vi "FPGA_DAQ_FixedPoint.vi"() -> ()   [LabVIEW 2019]
doc: "This VI provides a template for customizing a waveform acquisition using delta-sigma based NI C Series analog input smodules."
uses:
  <vilib>/LabVIEW Targets/FPGA/cRIO/shared/nicrio_ModuleControls/nicrio_cRIO-9219_ConversionTime.ctl
  <vilib>/rvi/Emulation/niFpgaSctlEmulationGetInTimedLoop.vi
  <vilib>/LabVIEW Targets/FPGA/cRIO/shared/nicrio_DsaDataRateApi/_nicrio_9225GetDataRate131.vi
  <vilib>/LabVIEW Targets/FPGA/cRIO/shared/nicrio_DsaDataRateApi/_nicrio_9234GetDataRate131.vi
  <vilib>/rvi/Emulation/niFpgaProcessEmulError.vi
  <vilib>/rvi/eio/common/nirviEmuTemplatePropertySet_errors.vi
  <vilib>/rvi/eio/common/nirviEmuTemplateMethod_errors.vi
  <vilib>/rvi/Emulation/niFpgaGetClockAttributes.vi
  <vilib>/rvi/Emulation/niFpgaEmulationReportErrorSimple.vi
  <vilib>/rvi/Emulation/niFpgaCriticalErrorInLSC.vi
  <vilib>/rvi/interface/RandomDataEmulation/niFpgaRandomDataHandleErrors.vi
  <vilib>/eio/EIOPropertyNode/EIOPropertyNode.xnode
  <vilib>/LabVIEW Targets/FPGA/cRIO/shared/nicrio_ModuleControls/nicrio_cRIO-9225_DataRatesRing.ctl
  <vilib>/LabVIEW Targets/FPGA/cRIO/shared/nicrio_ModuleControls/nicrio_cRIO-9234_DataRatesRing2.ctl
  <vilib>/eio/EIONode/EIONode.xnode
  <vilib>/rvi/DataTransferAndStorage/Container/XNode/niFpgaContainer.xnode
  <vilib>/rvi/interface/RandomDataEmulation/nirviRandomDataFpgaReadWriteTemplate.vi
  <vilib>/rvi/eio/common/nirviEmuTemplatePropertyGet_errors.vi
  <vilib>/rvi/eio/common/nirviEmuTemplatePropertyGet_noerrors.vi
  <vilib>/rvi/eio/common/nirviEmuTemplatePropertySet_noerrors.vi
panel:
  in  "Measurements per cycle":i16
  out "StopGeral":bool
  out "CJC1":fxp<+/-,32,-1>
  out "CJC0":fxp<+/-,32,-1>
  out "Temp3":fxp<+,32,14>
  out "Temp2":fxp<+,32,14>
  out "Temp1":fxp<+/-,32,-1>
  out "Temp0":fxp<+/-,32,-1>
  out "Ten oclk mult":u32
  out "Ten oclk div":u32
  out "Ten oclk freq":u32
  out "Vib oclk mult":u32
  out "Vib oclk div":u32
  out "Vib oclk freq":u32
  out "Acq Loop uS":u32
  out "FPGA Error":errorcluster
  out "Module Underflow":bool
  out "Finished":bool
  out "First Read":bool
  out "DMA FIFO Full":bool
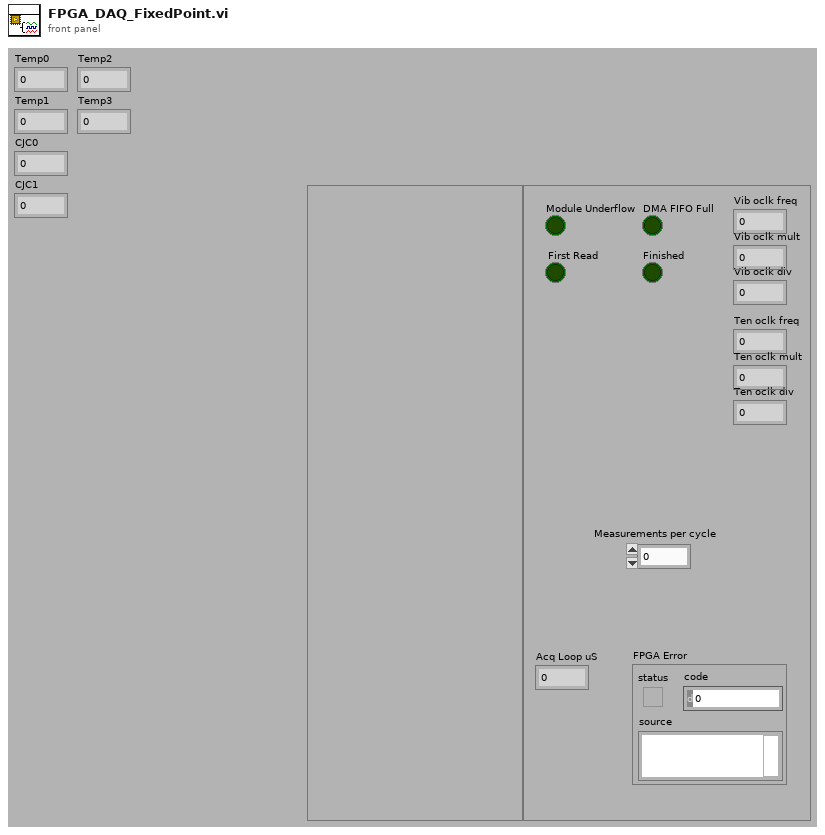
[diagram p1: front panel]
types:
  T1 = typedef "nicrio_cRIO-9219_ConversionTime.ctl" = enum8{"High Speed", "Best 60 Hz Rejection", "Best 50 Hz Rejection", "High Resolution"}
  T2 = typedef "nicrio_cRIO-9234_DataRatesRing2.ctl" = u8
  T3 = typedef "nicrio_cRIO-9225_DataRatesRing2.ctl" = u8
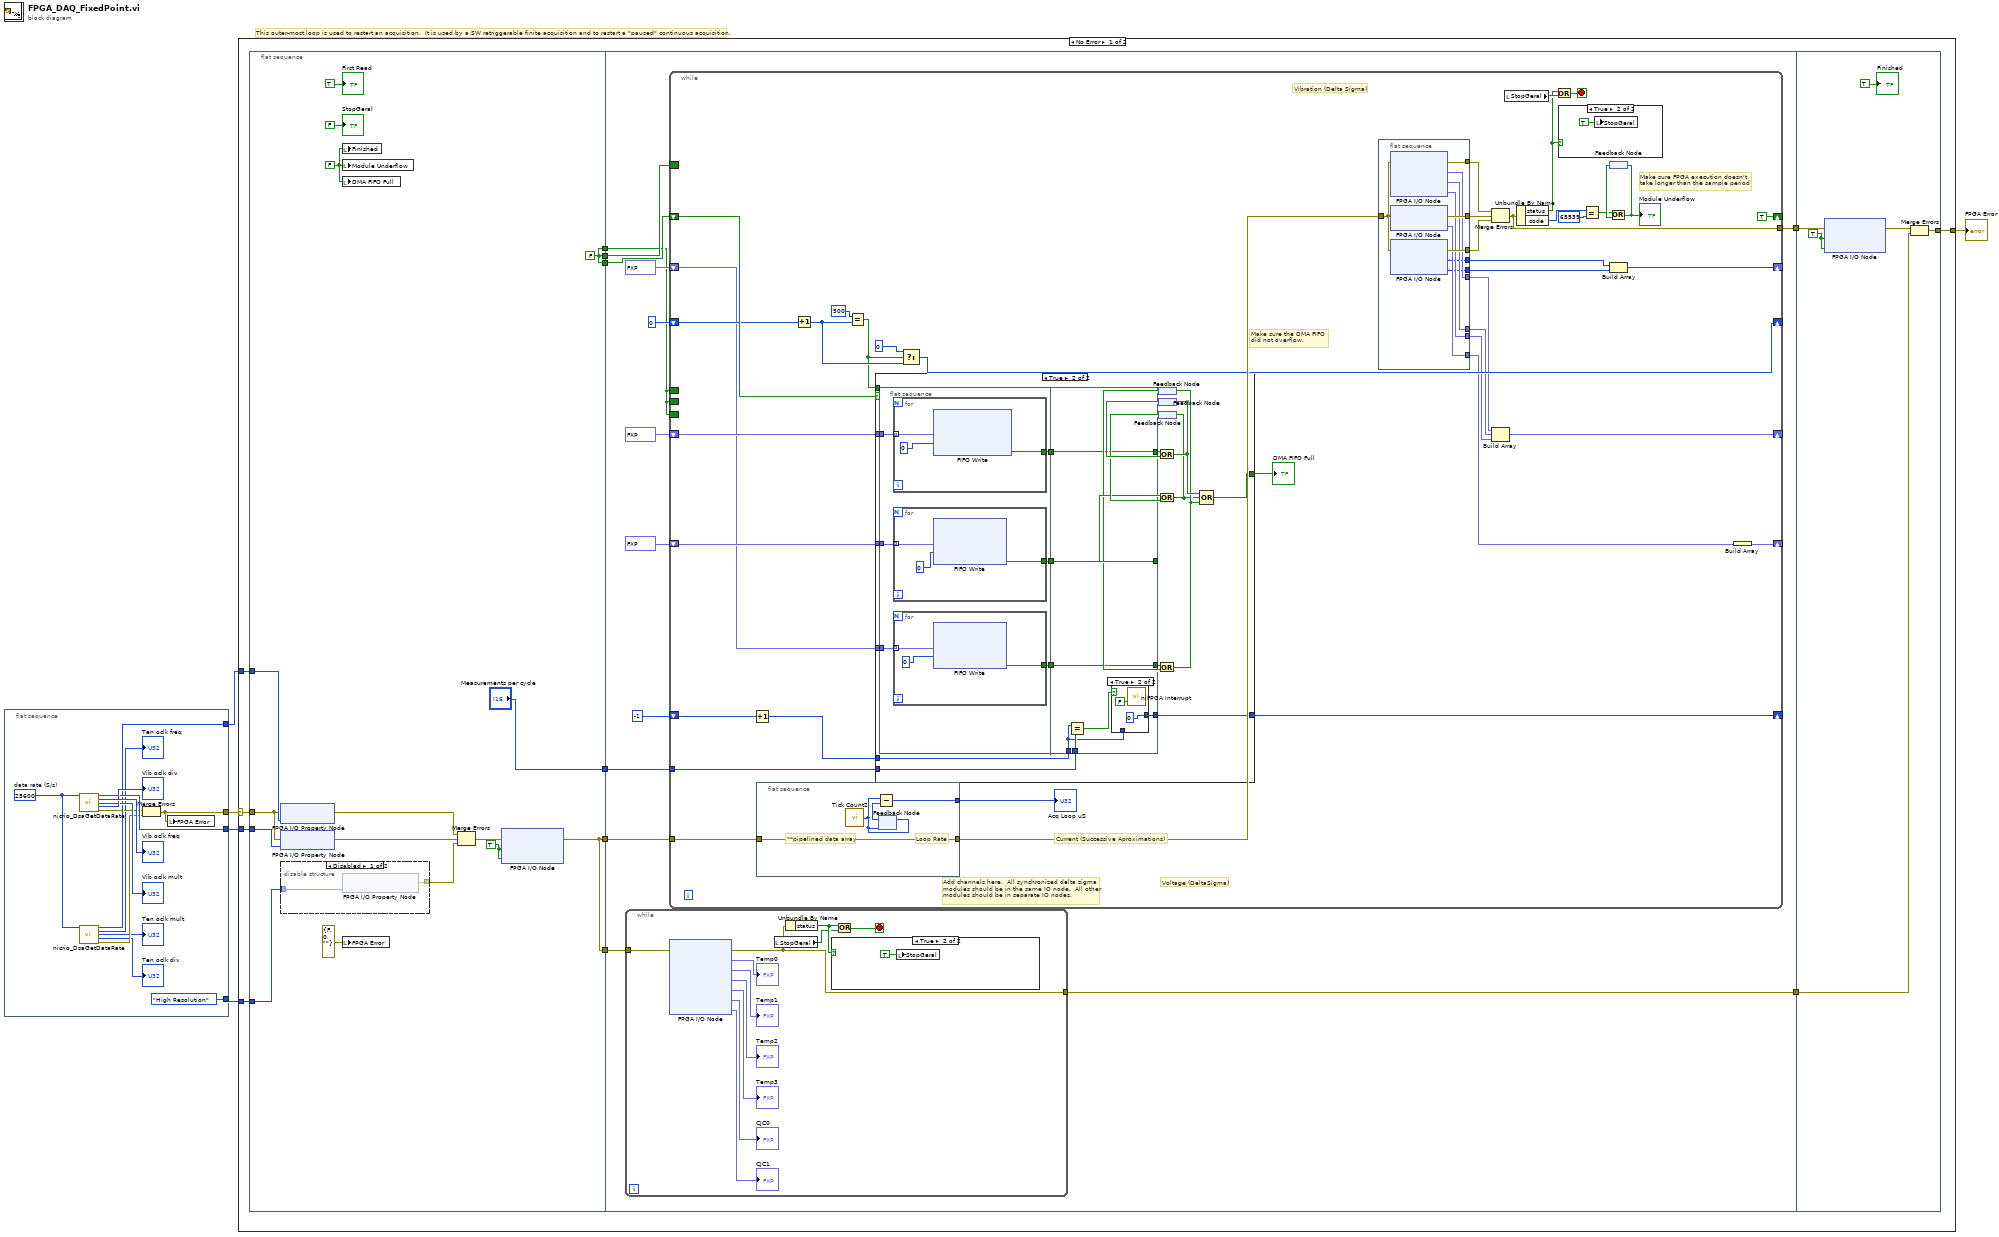
[diagram p0: block diagram]
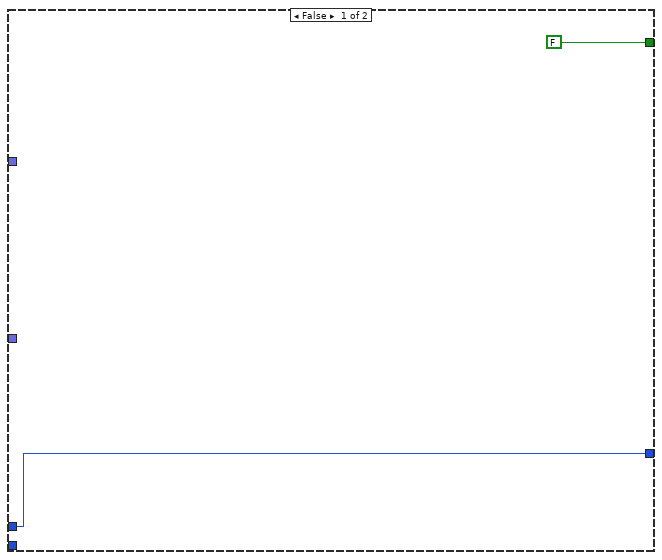
[diagram p5: hidden frame]
diagram:
  # "This outer-most loop is used to restart an acquisition.  It is used by a SW retriggerable finite acquisition and to restart a \"paused\" continuous acquisition."
  n1 = flat-sequence {
    tunnel: [w10] -> w3
    tunnel: [w15] -> w4
    tunnel: [w14] -> w2
    tunnel: [nicrio_cRIO-9219_ConversionTime."High Resolution" ("Conversion Time")] -> w1
    frame #0 {
      w13 = u32 25600  # data rate (S/s)
      n2 = call-poly <vilib>:"nicrio_DsaGetDataRate.vi"("data rate (S/s)"=w13) -> ("data rate"=w15:T2, "oclk freq"=→"Vib oclk freq":u32, "oclk mult"=→"Vib oclk mult":u32, "oclk div"=→"Vib oclk div":u32, "error out"=w12:errorcluster)  [unwired: 10 in]
      n3 = call-poly <vilib>:"nicrio_DsaGetDataRate.vi"("data rate (S/s)"=w13) -> ("data rate"=w14:T3, "oclk freq"=→"Ten oclk freq":u32, "oclk mult"=→"Ten oclk mult":u32, "oclk div"=→"Ten oclk div":u32, "error out"=w11:errorcluster)  [unwired: 10 in]
      n4 = Merge Errors(w12, w11) -> (w10:errorcluster)
      n5 = local write "FPGA Error"(w10) -> ()
    }
  }
  n6 = case shown="No Error" w3 {
    selector: w3 -> [w26 w182]
    tunnel: [w28 w182] -> w5
    tunnel: w4 -> [w27 _]
    tunnel: w2 -> [w23 _]
    tunnel: w1 -> [w21 _]
    frame No Error {
      n7 = flat-sequence {
        tunnel: [w36] -> w31
        tunnel: [w44] -> w30
        tunnel: w27 -> [w45]
        tunnel: w26 -> [w40]
        tunnel: [w44] -> w25
        tunnel: [w44] -> w24
        tunnel: w23 -> [w42]
        tunnel: [w36] -> w22
        tunnel: w21 -> [w35]
        tunnel: ["Measurements per cycle"] -> w19
        tunnel: w31 -> [w62]
        tunnel: [w60] -> w29
        tunnel: w30 -> [w52]
        tunnel: w25 -> [w59]
        tunnel: w24 -> [w61]
        tunnel: w22 -> [w58]
        tunnel: [w57] -> w20
        tunnel: w19 -> [w50]
        tunnel: w29 -> [w179]
        tunnel: [w177] -> w28
        tunnel: w20 -> [w176]
        frame #0 {
          w44 = FALSE
          w41 = FALSE ("Module Underflow")
          w43 = TRUE ("Mod1/Start")
          n8 = xnode "FPGA I/O Property Node"("error in"=w40, "Data Rate"=w42) -> ("error out"=w38:errorcluster)  [unwired: 1 in, 1 out]
          n9 = xnode "FPGA I/O Property Node"("error in"=w40, "Data Rate"=w45) -> ("error out"=w39:errorcluster)  [unwired: 1 in, 1 out]
          n10 = disable-structure shown="Disabled" {
            disable-tunnel: w35 -> [w49 _]
            disable-tunnel: [w48 _] -> w34
            frame Disabled {
              n11 = xnode "FPGA I/O Property Node"("Conversion Time"=w49) -> ("error out"=w48:errorcluster)  [unwired: 2 in, 1 out]
            }
            frame Enabled {
            }
          }
          n12 = local write "Finished"(w41) -> ()
          n13 = local write "Module Underflow"(w41) -> ()
          n14 = local write "DMA FIFO Full"(w41) -> ()
          n15 = local write "FPGA Error"(errorcluster {"status"=FALSE, "code"=0, "source"=""} ("FPGA Error")) -> ()
          n16 = Merge Errors(w38, w39, w34) -> (w37:errorcluster)
          n17 = xnode "FPGA I/O Node"("error in"=w37, "Mod3/Start"=w43, "Mod4/Start"=w43) -> ("error out"=w36:errorcluster)  [unwired: 2 in, 2 out]
          "First Read" <- TRUE ("First Read")
          "StopGeral" <- FALSE ("StopGeral")
        }
        frame #1 {
          n18 = while {
            tunnel: w58 -> [w67]
            tunnel: [w66] -> w57
            stop <- w63 stop-if-true
            n19 = xnode "FPGA I/O Node"("error in"=w67) -> ("error out"=w66:errorcluster, "Mod1/CH0"=→"Temp0":fxp<+/-,32,-1>, "Mod1/CH1"=→"Temp1":fxp<+/-,32,-1>, "Mod1/CH2"=→"Temp2":fxp<+,32,14>, "Mod1/CH3"=→"Temp3":fxp<+,32,14>, "Mod1/CJC0"=→"CJC0":fxp<+/-,32,-1>, "Mod1/CJC1"=→"CJC1":fxp<+/-,32,-1>)  [unwired: 6 in, 6 out]
            n20 = local read "StopGeral"() -> (w64:bool)
            n21 = Unbundle By Name(w66) -> ("status"=w65:bool)
            n22 = case shown="True" w65 {
              frame False {
              }
              frame True {
                n23 = local write "StopGeral"(TRUE ("StopGeral")) -> ()
              }
            }
            n24 = Or(x=w65, y=w64) -> (x .or. y?=w63:bool)
          }
          n25 = while {
            tunnel: w62 -> [w112]
            tunnel: [w101] -> w60
            shift-right: [TRUE ("t")] -> _
            shift-left: w61 -> [w110]
            border: w52 -> [_]
            border: w59 -> [_]
            shift-right: [w87] -> _
            shift-left: fxp<+/-,24,4>[] [0.0, 0.0, 0.0] -> [w97]
            shift-right: [w93] -> _
            shift-left: 0 ("Timeout") -> [w96]
            border: w52 -> [_]
            border: w52 -> [_]
            shift-right: [w85] -> _
            shift-left: fxp<+/-,24,10>[] [0.0] -> [w80]
            shift-right: [w81] -> _
            shift-left: fxp<+/-,20,5>[] [0.0, 0.0] -> [w79]
            shift-right: [w75] -> _
            shift-left: i16 -1 -> [w78]
            tunnel: w50 -> [w76]
            stop <- w99 stop-if-true
            # "Voltage (DeltaSigma)"
            # "Current (Successive Aproximations)"
            # "Vibration (Delta Sigma)"
            # "Add channels here.  All synchronized delta sigma\nmodules should be in the same IO node.  All other\nmodules should be in separate IO nodes."
            # "Make sure the DMA FIFO\ndid not overflow."
            # "Make sure FPGA execution doesn't\ntake longer than the sample period"
            n26 = Increment(x=w78) -> (x+1=w77:i16)
            n27 = flat-sequence {
              tunnel: [w175] -> w102
              tunnel: w112 -> [w175]
              tunnel: [w172] -> w111
              frame #0 {
                # "**pipelined data array"
                # "Loop Rate"
                n28 = call "Tick Count2"() -> ("Tick Count(uSec)"=w174:u32)
                n29 = feedback-in #1(w174) -> ()
                n30 = feedback #1(w174) -> (w173:u32)
                n31 = Subtract(x=w174, y=w173) -> (x-y=w172:u32)
              }
            }
            n32 = Increment(x=w96) -> (x+1=w94:i32)
            n33 = Equal?(x=500, y=w94) -> (x = y?=w91:bool)
            n34 = case shown="True" w110 {
              tunnel: [FALSE w145] -> w86
              tunnel: w97 -> [_ w146]
              tunnel: w91 -> [_ _]
              tunnel: w80 -> [_ w135]
              tunnel: w79 -> [_ w134]
              tunnel: w77 -> [w126 w130]
              tunnel: w76 -> [_ w129]
              tunnel: [w126 w128] -> w75
              frame False {
              }
              frame True {
                n35 = flat-sequence {
                  tunnel: w146 -> [w152]
                  tunnel: w135 -> [w148]
                  tunnel: w134 -> [w147]
                  tunnel: [w151] -> w133
                  tunnel: [w150] -> w132
                  tunnel: [w149] -> w131
                  tunnel: [w166] -> w136
                  tunnel: [w167] -> w140
                  tunnel: [w168] -> w142
                  tunnel: w133 -> [w168]
                  tunnel: w132 -> [w167]
                  tunnel: w131 -> [w166]
                  tunnel: w130 -> [w163]
                  tunnel: w129 -> [w165]
                  tunnel: [w162] -> w128
                  frame #0 {
                    n36 = for {
                      tunnel: [w161] -> w151
                      tunnel: w152 -> [w160] mode=indexing
                      n37 = xnode ("FIFO Write")("Element"=w160, "Timeout"=0) -> ("Timed Out?"=w161:bool)  [unwired: 1 in, 1 out]
                    }
                    n38 = for {
                      tunnel: [w158] -> w150
                      tunnel: w148 -> [w157] mode=indexing
                      n39 = xnode ("FIFO Write")("Element"=w157, "Timeout"=0) -> ("Timed Out?"=w158:bool)  [unwired: 1 in, 1 out]
                    }
                    n40 = for {
                      tunnel: [w155] -> w149
                      tunnel: w147 -> [w154] mode=indexing
                      n41 = xnode ("FIFO Write")("Element"=w154, "Timeout"=0) -> ("Timed Out?"=w155:bool)  [unwired: 1 in, 1 out]
                    }
                  }
                  frame #1 {
                    n42 = Equal?(x=w163, y=w165) -> (x = y?=w164:bool)
                    n43 = case shown="True" w164 {
                      tunnel: w163 -> [w169 _]
                      tunnel: [w169 i16 0] -> w162
                      frame False {
                      }
                      frame True {
                        n44 = call <vilib>:"niFPGA Interrupt.vi"("Wait Until Cleared (F)"=FALSE) -> ()  [unwired: 2 in]
                      }
                    }
                  }
                }
                n45 = feedback #2() -> (w137:bool)
                n46 = Or(x=w136, y=w137) -> (x .or. y?=w139:bool)
                n47 = feedback-in #2(w139) -> ()
                n48 = feedback #3() -> (w143:bool)
                n49 = Or(x=w142, y=w143) -> (x .or. y?=w144:bool)
                n50 = feedback-in #3(w144) -> ()
                n51 = feedback #4() -> (w141:bool)
                n52 = Or(x=w140, y=w141) -> (x .or. y?=w138:bool)
                n53 = feedback-in #4(w138) -> ()
                n54 = Compound Arithmetic op=OR(w144, w138, w139) -> (w145:bool)
              }
            }
            "DMA FIFO Full" <- w86
            n55 = Select(t=u16 0, s=w91, f=w94) -> (s? t:f=w93:i32)
            n56 = flat-sequence {
              tunnel: [w124] -> w105
              tunnel: [w123] -> w104
              tunnel: [w122] -> w103
              tunnel: w102 -> [w121]
              tunnel: [w120] -> w90
              tunnel: [w119] -> w89
              tunnel: [w118] -> w88
              tunnel: [w117] -> w84
              tunnel: [w116] -> w83
              tunnel: [w115] -> w82
              frame #0 {
                n57 = xnode "FPGA I/O Node"("error in"=w121) -> ("error out"=w124:errorcluster, "Mod3/AI0"=w120:fxp<+/-,24,4>, "Mod3/AI1"=w119:fxp<+/-,24,4>, "Mod3/AI2"=w118:fxp<+/-,24,4>)  [unwired: 3 in, 3 out]
                n58 = xnode "FPGA I/O Node"("error in"=w121) -> ("error out"=w123:errorcluster, "Mod4/AI0"=w117:fxp<+/-,24,10>)  [unwired: 1 in, 1 out]
                n59 = xnode "FPGA I/O Node"("error in"=w121) -> ("error out"=w122:errorcluster, "Mod2/AI0"=w116:i16, "Mod2/AI1"=w115:i16)  [unwired: 2 in, 2 out]
              }
            }
            n60 = Merge Errors(w105, w104, w103) -> (w101:errorcluster)
            n61 = Build Array(w90, w89, w88) -> (w87:fxp<+/-,24,4>[])
            n62 = local read "StopGeral"() -> (w100:bool)
            n63 = Unbundle By Name(w101) -> ("status"=w98:bool, "code"=w113:i32)
            n64 = Or(x=w98, y=w100) -> (x .or. y?=w99:bool)
            n65 = case shown="True" w98 {
              frame False {
              }
              frame True {
                n66 = local write "StopGeral"(TRUE ("StopGeral")) -> ()
              }
            }
            n67 = Equal?(x=w113, y=65539) -> (x = y?=w107:bool)
            n68 = feedback #5() -> (w108:bool)
            n69 = Or(x=w107, y=w108) -> (x .or. y?=w106:bool)
            "Module Underflow" <- w106
            n70 = feedback-in #5(w106) -> ()
            n71 = Build Array(w83, w82) -> (w81:i16[])
            n72 = Build Array(w84) -> (w85:fxp<+/-,24,10>[])
            "Acq Loop uS" <- w111
          }
        }
        frame #2 {
          w180 = TRUE ("Mod1/Stop")
          n73 = xnode "FPGA I/O Node"("error in"=w179, "Mod3/Stop"=w180, "Mod4/Stop"=w180) -> ("error out"=w178:errorcluster)  [unwired: 2 in, 2 out]
          n74 = Merge Errors(w178, w176) -> (w177:errorcluster)
          "Finished" <- TRUE ("Finished")
        }
      }
    }
    frame Error {
    }
  }
  "FPGA Error" <- w5
